vi "_emi_SMLoop Get State Single.vi"(5 "Loop ID in":u16, 9 "error in (no error)":errorcluster) -> (1 "Enabled, not running, trice":bool, 2 "Enabled, not running, twice":bool, 3 "Enabled, not running":bool, 6 "Loop ID out":u16, 8 "Loop Running Out":bool, 10 "error out":errorcluster, 14 "Loop Enable Out":bool)   [LabVIEW 2011]
doc: "Retreive the execution state of the loop designated by Index. Used to syncronice different loops in teh same master loop.\n\nTo discover if the loop is failing to start, or has stopped unnececerily, check if \"Enabled, not running, twice \" or Trice is True. (Once can easily detect delay between Enablke and start). Distance between calls needs to be greater then the SMLoops Standby time."
uses:
  Loop control/Private/_emi_Loop control int action.ctl
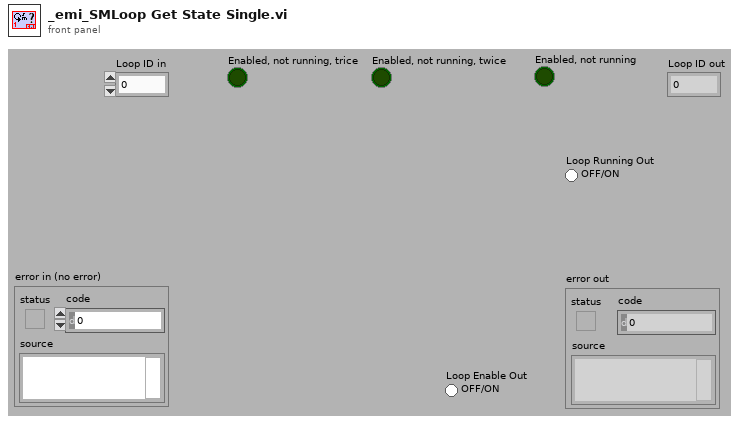
[diagram p1: front panel]
types:
  T1 = typedef "_emi_Loop control int action.ctl" = enum16{"Init index", "Get index", "Set index", "Get Size"}
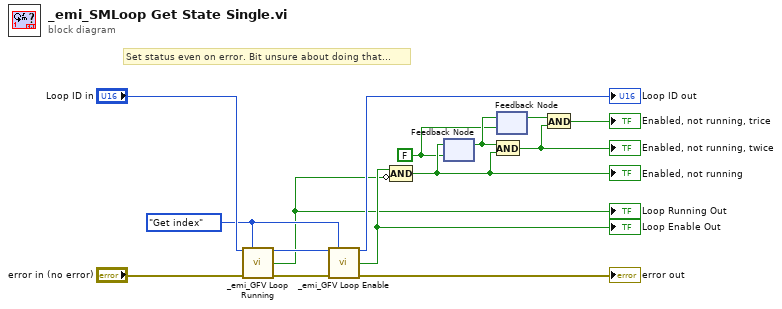
[diagram p0: block diagram]
diagram:
  w1 = FALSE
  w11 = _emi_Loop_control_int_action."Get index" ("Action(Get Index)")
  # "Set status even on error. Bit unsure about doing that..."
  n1 = call "_emi_GFV Loop Running.vi"("Loop Index/Numb"="Loop ID in", "Action(Get Index)"=w11, "error in (no error)"="error in (no error)") -> ("Index out"=w10:u16, "Loop Running Out"=w7:bool, "error out"=w13:errorcluster)  [unwired: 9 in, 1 out]
  "Loop Running Out" <- w7
  n2 = call "_emi_GFV Loop Enable.vi"("Loop Index/Numb"=w10, "Action(Get Index)"=w11, "error in (no error)"=w13) -> ("Index out"=→"Loop ID out":u16, "Loop Enable Out"=w8:bool, "error out"=→"error out":errorcluster)  [unwired: 9 in, 1 out]
  "Loop Enable Out" <- w8
  n3 = Compound Arithmetic op=AND(w8, invert w7) -> (w6:bool)
  "Enabled, not running" <- w6
  n4 = feedback-in #1(w6) -> ()
  n5 = feedback #1(w1) -> (w5:bool)
  n6 = And(x=w5, y=w6) -> (x .and. y?=w3:bool)
  "Enabled, not running, twice" <- w3
  n7 = feedback #2(w1) -> (w4:bool)
  n8 = feedback-in #2(w5) -> ()
  n9 = And(x=w4, y=w3) -> (x .and. y?=→"Enabled, not running, trice":bool)
